vi "Delete Recursive__ogtk.vi"(8 "error in (no error)":errorcluster, 9 "Ignore Read-Only? (FALSE)":bool, 10 "Recursive? (FALSE)":bool, 11 "Path":path) -> (0 "error out":errorcluster, 3 "dup Path":path)   [LabVIEW 2009]
doc: "Deletes the file or directory specified by path. If path specifies a directory that is not empty and \"Recursive\" is FALSE or if you do not have write permission for both the file or directory specified by path and its parent directory and \"Ignore Read-Only\" is FALSE, this function does not remove the directory and returns an error."
uses:
  Build Path - File Names Array__ogtk.vi
panel:
  # "Delete Recursive.vi\n\nCan deletes all files and subfolders of a folder\n\nPlease visit http://www.OpenG.org to learn about the\nOpen Source LabVIEW software movement.\n\nNOTICE -- YOU MUST LEAVE THIS NOTICE IN PLACE.  PER THE TERMS OF THE LICENSE BELOW, YOU MAY SUBLICENSE THIS SOFTWARE \nIN ANY WAY THAT DOES NOT CONFLICT WITH THIS LICENSE.\n\n### BSD License (http://www.opensource.org/licenses/bsd-license.php) Begin ###\n\nCopyright (c) 2006, JKI <info@jameskring.com>\nCopyright (c) 2002, Jim Kring <jim@jimkring.com>\nCopyright (c) 2002, Cal-Bay Systems, Inc. <info@calbay.com>\n\nAll rights reserved.\n\nRedistribution and use in source and binary forms, with or without modification, are permitted provided that the following conditions are met:\n\n    * Redistributions of source code must retain the above copyright notice, this list of conditions and the following disclaimer.\n    * Redistributions in binary form must reproduce the above copyright notice, this list of conditions and the following disclaimer in the \n       documentation and/or other materials provided with the distribution.\n    * Neither the name of SciWare, James Kring, Inc., nor the names of its contributors may be used to endorse or promote products derived \n       from this software without specific prior written permission.\n\nTHIS SOFTWARE IS PROVIDED BY THE COPYRIGHT HOLDERS AND CONTRIBUTORS \"AS IS\" AND ANY EXPRESS OR IMPLIED WARRANTIES, \nINCLUDING, BUT NOT LIMITED TO, THE IMPLIED WARRANTIES OF MERCHANTABILITY AND FITNESS FOR A PARTICULAR PURPOSE ARE \nDISCLAIMED. IN NO EVENT SHALL THE COPYRIGHT OWNER OR CONTRIBUTORS BE LIABLE FOR ANY DIRECT, INDIRECT, INCIDENTAL,\n SPECIAL, EXEMPLARY, OR CONSEQUENTIAL DAMAGES (INCLUDING, BUT NOT LIMITED TO, PROCUREMENT OF SUBSTITUTE GOODS OR \nSERVICES; LOSS OF USE, DATA, OR PROFITS; OR BUSINESS INTERRUPTION) HOWEVER CAUSED AND ON ANY THEORY OF LIABILITY, \nWHETHER IN CONTRACT, STRICT LIABILITY, OR TORT (INCLUDING NEGLIGENCE OR OTHERWISE) ARISING IN ANY WAY OUT OF THE USE \nOF THIS SOFTWARE, EVEN IF ADVISED OF THE POSSIBILITY OF SUCH DAMAGE.\n\n### BSD License End ###"
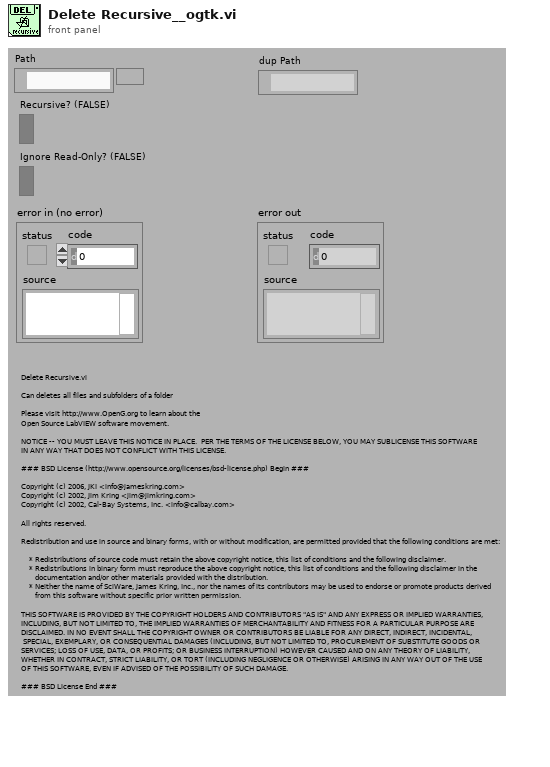
[diagram p1: front panel]
types:
  T1 = cluster{"Archive":bool, "Normal":bool, "Temporary":bool, "Compressed":bool, "Offline":bool, "Content Indexed":bool, "Encrypted (cannot set)":bool}
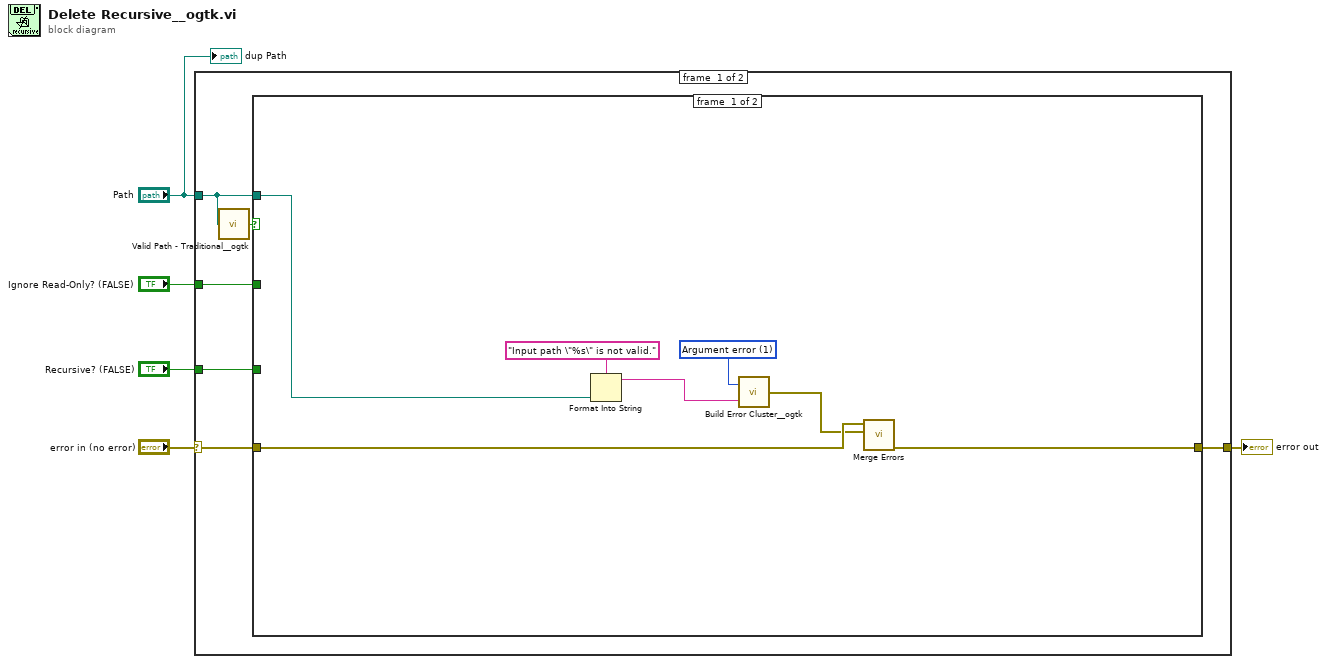
[diagram p0: block diagram]
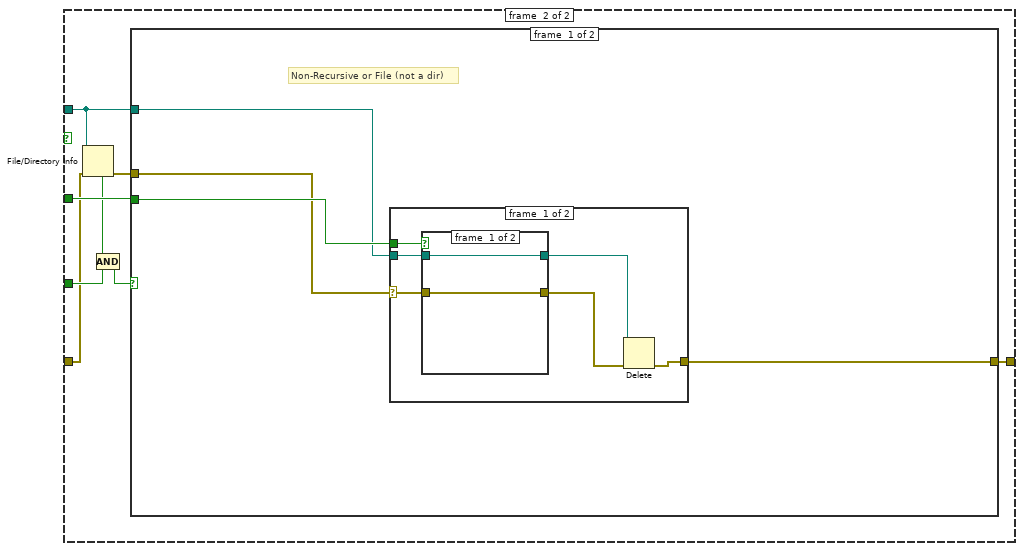
[diagram p2: hidden frame]
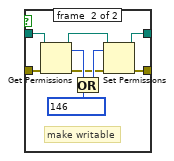
[diagram p3: hidden frame]
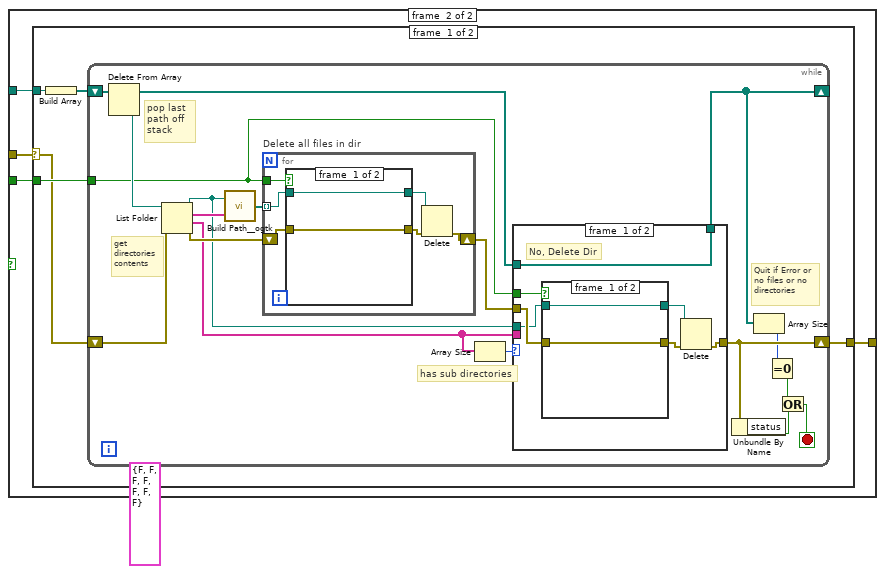
[diagram p5: hidden frame]
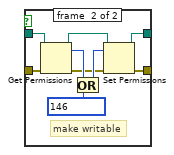
[diagram p6: hidden frame]
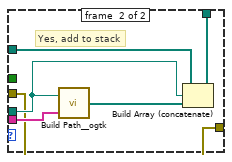
[diagram p7: hidden frame]
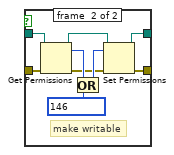
[diagram p8: hidden frame]
diagram:
  n1 = case shown="No Error" "error in (no error)" {
    selector: "error in (no error)" -> [w6 w118]
    tunnel: "Ignore Read-Only? (FALSE)" -> [w11 _]
    tunnel: [w10 w118] -> w4
    tunnel: "Recursive? (FALSE)" -> [w9 _]
    tunnel: "Path" -> [w8 _]
    frame #0 {
      n2 = call "Valid Path - Traditional__ogtk.vi"("path"=w8) -> ("valid"=w7:bool)
      n3 = case shown="True" w7 {
        tunnel: w11 -> [_ w26]
        tunnel: [w18 w25] -> w10
        tunnel: w8 -> [w14 w24]
        tunnel: w9 -> [_ w22]
        tunnel: w6 -> [w17 w20]
        frame #0 {
          w16 = 1 items=["No error", "Argument error", "Memory is full", "Out of zone", "End of file", "File already open", "Generic file I/O error", "File not found", "File permission error", "Disk is full", "Duplicate path", "Too many files open", "System feature not enabled", "Resource file not found", "Cannot add resource", "Resource not found", "Image not found", "Image memory error", "Pen does not exist", "Config type invalid", "Config token not found", "Config parse error", "Config memory error", "Bad external code format", "Bad external code offset", "External code not present", "Null window", "Destroy window error", "Null menu", "Print aborted", "Bad print record", "Print driver error", "Windows error during printing", "Memory error during printing", "Print dialog error", "Generic print error", "Invalid device refnum", "Device not found", "Device parameter error", "Device unit error", "Cannot open device", "Device call aborted", "Generic error", "Cancelled by user", "Object ID too low", "Object ID too high", "Object not in heap", "Unknown heap", "Unknown object (invalid DefProc)", "Unknown object (DefProc not in table)", "Message out of range", "Invalid (null) method", "Unknown message", "Manager call not supported", "Bad address", "Network operation in progress", "Network operation timed out", "Connection is busy", "Network attribute not supported", "Network error", "Address in use", "System out of memory", "Connection aborted", "Connection refused", "Not connected", "Already connected", "Connection closed", "Initialization error (interapplication manager)", "Bad occurrence", "Wait on unbound occurrence handler", "Occurrence queue overflow", "Datalog type conflict", "Unused", "Unrecognized type (interapplication manager)", "Memory corrupt", "Failed to make temporary DLL", "Old CIN version", "Drag socket not found", "Failed to load drop-object", "Failed to register OLE object", "Failed to release OLE object", "Format specifier type mismatch", "Unknown format specifier", "Too few format specifiers", "Too many format specifiers", "Scan failed", "Newer CIN version", "Error converting to variant", "Runtime menu error", "Password tampered", "Variant attribute not found", "Incompatible variant data type", "Event data is not available", "Event Store is not present", "Occurrence is not found", "Event Queue is not created", "Event info is not available", "Refnum passed is NULL", "Error retrieving Class GUID", "Error retrieving CoClass GUID", "Error retrieving TypeLib GUID.", "Bad built application magic bytes.", "Specific driver is different from the specific driver associated with the Logical Name.", "There is no session opened to the class driver.", "Max Error", "MAX - Error with config objects", "MAX - Error loading configuration", "MAX - Group not supported"]
          n4 = Format Into String(format string="Input path \"%s\" is not valid.", w14) -> (resulting string=w12:string)  [unwired: 2 in, 1 out]
          n5 = call <userlib>:"Build Error Cluster__ogtk.vi"("String to Prepend to source (\"\")"=w12, "code"=w16) -> ("error out"=w15:errorcluster)
          n6 = call <vilib>:"Merge Errors.vi"("error in 2 (no error)"=w15, "error in 1 (no error)"=w17) -> ("error out"=w18:errorcluster)  [unwired: 5 in]
        }
        frame #1 {
          n7 = File/Directory Info(path=w24, error in=w20) -> (directory=w23:bool, error out=w19:errorcluster)  [unwired: 5 out]
          n8 = Compound Arithmetic op=AND(w23, w22) -> (w21:bool)
          n9 = case shown="True" w21 {
            tunnel: w19 -> [w27 w49]
            tunnel: [w30 w52] -> w25
            tunnel: w24 -> [w28 w50]
            tunnel: w26 -> [w29 w51]
            frame #0 {
              # "Non-Recursive or File (not a dir)"
              n10 = case shown="No Error" w27 {
                selector: w27 -> [w31 w48]
                tunnel: [w36 w48] -> w30
                tunnel: w29 -> [w35 _]
                tunnel: w28 -> [w34 _]
                frame #0 {
                  n11 = case shown="True" w35 {
                    tunnel: w31 -> [w37 w42]
                    tunnel: [w37 w41] -> w32
                    tunnel: [w38 w40] -> w33
                    tunnel: w34 -> [w38 w39]
                    frame #0 {
                    }
                    frame #1 {
                      # "make writable"
                      n12 = Get Permissions(8:w42, 11:w39) -> (0:w43:errorcluster, 3:w45:path, 5:w47:i16)  [unwired: 2 out]
                      n13 = Or(x=w47, y=i16 146 ("Read Only")) -> (x .or. y?=w44:i16)
                      n14 = Set Permissions(7:w44, 8:w43, 11:w45) -> (0:w41:errorcluster, 3:w40:path)  [unwired: 2 in]
                    }
                  }
                  n15 = Delete(path (use dialog)=w33, error in=w32) -> (error out=w36:errorcluster)  [unwired: 3 in, 2 out]
                }
                frame #1 {
                }
              }
            }
            frame #1 {
              n16 = case shown="No Error" w49 {
                selector: w49 -> [w54 w117]
                tunnel: [w57 w117] -> w52
                tunnel: w51 -> [w56 _]
                tunnel: w50 -> [w55 _]
                frame #0 {
                  n17 = Build Array(w55) -> (w53:path[])
                  n18 = while {
                    shift-right: [w64] -> _
                    shift-left: w53 -> [w65]
                    shift-right: [w71] -> w57
                    shift-left: w54 -> [w66]
                    tunnel: w56 -> [w58]
                    stop <- w67 stop-if-true
                    (unwired) T1 {"Archive"=FALSE, "Normal"=FALSE, "Temporary"=FALSE, "Compressed"=FALSE, "Offline"=FALSE, "Content Indexed"=FALSE, "Encrypted (cannot set)"=FALSE} ("FileAttribute")
                    # "get directories contents"
                    # "pop last path off stack"
                    # "Quit if Error or no files or no directories"
                    # "has sub directories"
                    n19 = Delete From Array(array=w65) -> (deleted portion=w59:path, array with subset deleted=w60:path[])  [unwired: 2 in]
                    n20 = List Folder(path=w59, error in=w66) -> (path out=w62:path, filenames=w63:string[], folder names=w72:string[], error out=w75:errorcluster)  [unwired: 2 in]
                    n21 = call-poly "Build Path__ogtk.vi"("name or relative path"=w63, "base path"=w62) -> ("appended path"=w61:path[])
                    n22 = for "Delete all files in dir" {
                      shift-right: [w105] -> w73
                      shift-left: w75 -> [w104]
                      tunnel: w58 -> [w101]
                      tunnel: w61 -> [w100] mode=indexing
                      n23 = case shown="True" w101 {
                        tunnel: w104 -> [w106 w111]
                        tunnel: [w106 w110] -> w103
                        tunnel: [w107 w109] -> w102
                        tunnel: w100 -> [w107 w108]
                        frame #0 {
                        }
                        frame #1 {
                          # "make writable"
                          n24 = Get Permissions(8:w111, 11:w108) -> (0:w112:errorcluster, 3:w114:path, 5:w116:i16)  [unwired: 2 out]
                          n25 = Or(x=w116, y=i16 146 ("Read Only")) -> (x .or. y?=w113:i16)
                          n26 = Set Permissions(7:w113, 8:w112, 11:w114) -> (0:w110:errorcluster, 3:w109:path)  [unwired: 2 in]
                        }
                      }
                      n27 = Delete(path (use dialog)=w102, error in=w103) -> (error out=w105:errorcluster)  [unwired: 3 in, 2 out]
                    }
                    n28 = Array Size(array=w72) -> (size(s)=w74:i32)
                    n29 = case shown="0" w74 {
                      tunnel: w62 -> [w77 w97]
                      tunnel: w73 -> [w79 w95]
                      tunnel: [w78 w95] -> w71
                      tunnel: w72 -> [_ w99]
                      tunnel: w60 -> [w82 w96]
                      tunnel: [w82 w94] -> w64
                      tunnel: w58 -> [w76 _]
                      frame #0 {
                        # "No, Delete Dir"
                        n30 = case shown="True" w76 {
                          tunnel: w79 -> [w83 w88]
                          tunnel: [w83 w87] -> w81
                          tunnel: [w84 w86] -> w80
                          tunnel: w77 -> [w84 w85]
                          frame #0 {
                          }
                          frame #1 {
                            # "make writable"
                            n31 = Get Permissions(8:w88, 11:w85) -> (0:w89:errorcluster, 3:w91:path, 5:w93:i16)  [unwired: 2 out]
                            n32 = Or(x=w93, y=i16 146 ("Read Only")) -> (x .or. y?=w90:i16)
                            n33 = Set Permissions(7:w90, 8:w89, 11:w91) -> (0:w87:errorcluster, 3:w86:path)  [unwired: 2 in]
                          }
                        }
                        n34 = Delete(path (use dialog)=w80, error in=w81) -> (error out=w78:errorcluster)  [unwired: 3 in, 2 out]
                      }
                      frame #1 {
                        # "Yes, add to stack"
                        n35 = call-poly "Build Path__ogtk.vi"("name or relative path"=w99, "base path"=w97) -> ("appended path"=w98:path[])
                        n36 = Build Array (concatenate)(w96, w97, w98) -> (w94:path[])
                      }
                    }
                    n37 = Unbundle By Name(w71) -> ("status"=w69:bool)
                    n38 = Array Size(array=w64) -> (size(s)=w70:i32)
                    n39 = Equal To 0?(x=w70) -> (x = 0?=w68:bool)
                    n40 = Or(x=w68, y=w69) -> (x .or. y?=w67:bool)
                  }
                }
                frame #1 {
                }
              }
            }
          }
        }
      }
    }
    frame #1 {
    }
  }
  "error out" <- w4
  "dup Path" <- "Path"
